vi "Motor&Controller test sequence.vi"() -> ()   [LabVIEW 2016]
uses:
  Set Save Object Dictionary.vi
  <vilib>/CANopenLib/CANOPEN.llb/CANopen SDO Create.vi
  Set mode of operation.vi
  <vilib>/CANopenLib/CANOPEN.llb/CANopen SDO Write.vi
  <vilib>/CANopenLib/CANOPEN.llb/CANopen SDO Write [STR].vi
  Get mode of operation.vi
  Set control mode.vi
  Set into drive mode.vi
  Set target speed.vi
  <vilib>/CANopenLib/CANOPEN.llb/CANopen SDO Close.vi
  <vilib>/CANopenLib/CANOPEN.llb/CANopen Interface Close.vi
panel:
  in  "OK Button":bool
  out "Mode of operation":i8(ring) items=["Induction VF – testing purposes only"=-5, "Aligning rotor position"=-4, "Current stepper – testing purposes only "=-3, "Voltage stepper – testing purposes only"=-2, "Voltage constant angle – testing purposes only"=-1, "No mode"=0, "Cyclic sync position"=8, "Cyclic sync velocity"=9, "Cyclic sync torque"=10]
  out "Error":errorcluster
  in  "Stop Button":bool
  in  "Motor Speed":i32(knob) min=0 max=1500 step=100 scale=0.0..2000.0
  in  "Motor":u8(ring) items=["Right", "Left"]
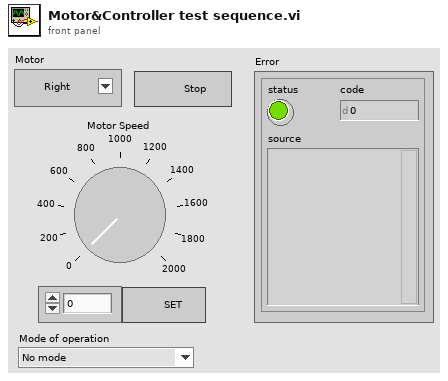
[diagram p1: front panel]
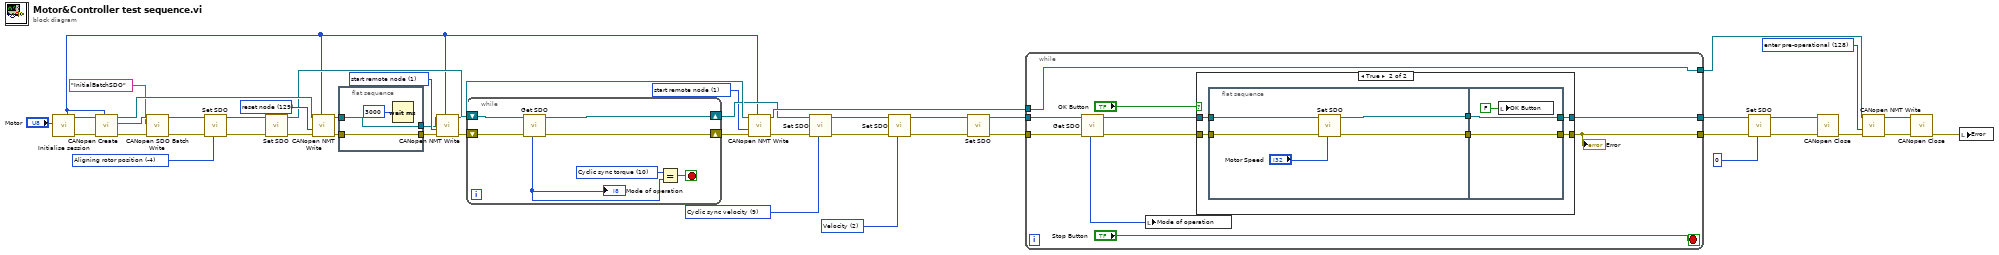
[diagram p0: block diagram]
diagram:
  w7 = u16 1 items=["start remote node"=1, "stop remote node"=2, "enter pre-operational"=128, "reset node"=129, "reset communication"=130] ("command")
  w15 = i8 9 items=["Induction VF – testing purposes only"=-5, "Aligning rotor position"=-4, "Current stepper – testing purposes only "=-3, "Voltage stepper – testing purposes only"=-2, "Voltage constant angle – testing purposes only"=-1, "No mode"=0, "Cyclic sync position"=8, "Cyclic sync velocity"=9, "Cyclic sync torque"=10] ("Mode of operation")
  w20 = u8 2 items=["Velocity"=2, "Torque"=1] ("Control Mode")
  w31 = u16 1 items=["start remote node"=1, "stop remote node"=2, "enter pre-operational"=128, "reset node"=129, "reset communication"=130] ("command")
  w32 = u16 129 items=["start remote node"=1, "stop remote node"=2, "enter pre-operational"=128, "reset node"=129, "reset communication"=130] ("command")
  w42 = u16 128 items=["start remote node"=1, "stop remote node"=2, "enter pre-operational"=128, "reset node"=129, "reset communication"=130] ("command")
  w46 = i8 -4 items=["Induction VF – testing purposes only"=-5, "Aligning rotor position"=-4, "Current stepper – testing purposes only "=-3, "Voltage stepper – testing purposes only"=-2, "Voltage constant angle – testing purposes only"=-1, "No mode"=0, "Cyclic sync position"=8, "Cyclic sync velocity"=9, "Cyclic sync torque"=10] ("Mode of operation")
  n1 = call "Initialise session.vi"("Motor"="Motor") -> ("error out"=w45:errorcluster, "interface object out"=w44:refnum<k20>, "Used Node ID"=w1:u8)  [unwired: 8 in]
  n2 = call-poly <vilib>:"CANopen Create.vi"("node-ID"=w1, "error in (no error)"=w45, "interface object in"=w44) -> ("error out"=w6:errorcluster, "SDO object out"=w3:refnum<k20>, "interface object out"=w27:refnum<k20>)  [unwired: 6 in]
  n3 = call <vilib>:"CANopen SDO Batch Write.vi"("error in (no error)"=w6, "batch SDO name"="InitialBatchSDO", "SDO object in"=w3) -> ("error out"=w5:errorcluster, "SDO object out"=w4:refnum<k20>)  [unwired: 6 in, 1 out]
  n4 = call-poly "Set SDO.vi"("Mode of operation"=w46, "error in (no error)"=w5, "SDO object in"=w4) -> ("error out"=w29:errorcluster, "SDO object out"=w30:refnum<k20>)  [unwired: 6 in, 1 out]
  n5 = call-poly "Set SDO.vi"("error in (no error)"=w29, "SDO object in"=w30) -> ("error out"=w28:errorcluster, "SDO object out"=w25:refnum<k20>)  [unwired: 7 in, 1 out]
  n6 = call <vilib>:"CANopen NMT Write.vi"("node-ID (0)"=w1, "error in (no error)"=w28, "command"=w32, "interface object in"=w27) -> ("error out"=w23:errorcluster, "interface object out"=w24:refnum<k20>)  [unwired: 6 in]
  n7 = flat-sequence {
    tunnel: w24 -> [w49]
    tunnel: w23 -> [w50]
    tunnel: [w50] -> w22
    tunnel: [w49] -> w21
    frame #0 {
      n8 = Wait (ms)(milliseconds to wait=u32 3000) -> ()  [unwired: 1 out]
    }
  }
  n9 = call <vilib>:"CANopen NMT Write.vi"("node-ID (0)"=w1, "error in (no error)"=w22, "command"=w31, "interface object in"=w21) -> ("error out"=w26:errorcluster, "interface object out"=w11:refnum<k20>)  [unwired: 6 in]
  n10 = while {
    shift-right: [w54] -> w12
    shift-left: w26 -> [w57]
    shift-right: [w55] -> w9
    shift-left: w25 -> [w56]
    stop <- w51 stop-if-true
    w53 = i8 10 items=["Induction VF – testing purposes only"=-5, "Aligning rotor position"=-4, "Current stepper – testing purposes only "=-3, "Voltage stepper – testing purposes only"=-2, "Voltage constant angle – testing purposes only"=-1, "No mode"=0, "Cyclic sync position"=8, "Cyclic sync velocity"=9, "Cyclic sync torque"=10] ("Mode of operation")
    n11 = call-poly "Get SDO.vi"("error in (no error)"=w57, "SDO object in"=w56) -> ("error out"=w54:errorcluster, "SDO object out"=w55:refnum<k20>, "Mode of operation"=w52:i8)  [unwired: 6 in, 1 out]
    "Mode of operation" <- w52
    n12 = Equal?(x=w53, y=w52) -> (x = y?=w51:bool)
  }
  n13 = call <vilib>:"CANopen NMT Write.vi"("node-ID (0)"=w1, "error in (no error)"=w12, "command"=w7, "interface object in"=w11) -> ("error out"=w8:errorcluster, "interface object out"=w10:refnum<k20>)  [unwired: 6 in]
  n14 = call-poly "Set SDO.vi"("Mode of operation"=w15, "error in (no error)"=w8, "SDO object in"=w9) -> ("error out"=w18:errorcluster, "SDO object out"=w19:refnum<k20>)  [unwired: 6 in, 1 out]
  n15 = call-poly "Set SDO.vi"("Control Mode"=w20, "error in (no error)"=w18, "SDO object in"=w19) -> ("error out"=w16:errorcluster, "SDO object out"=w17:refnum<k20>)  [unwired: 6 in, 1 out]
  n16 = call-poly "Set SDO.vi"("error in (no error)"=w16, "SDO object in"=w17) -> ("error out"=w13:errorcluster, "SDO object out"=w14:refnum<k20>)  [unwired: 8 in]
  n17 = while {
    tunnel: [w66] -> w41
    tunnel: [w64] -> w40
    tunnel: w10 -> [w65]
    tunnel: [w65] -> w39
    tunnel: w14 -> [w59]
    tunnel: w13 -> [w58]
    stop <- "Stop Button" stop-if-true
    n18 = call-poly "Get SDO.vi"("error in (no error)"=w58, "SDO object in"=w59) -> ("error out"=w60:errorcluster, "SDO object out"=w61:refnum<k20>, "Mode of operation"=w62:i8)  [unwired: 6 in, 1 out]
    n19 = local write "Mode of operation"(w62) -> ()
    n20 = case shown="True" "OK Button" {
      tunnel: [w69 w75] -> w66
      tunnel: [w68 w74] -> w64
      tunnel: w61 -> [w69 w71]
      tunnel: w60 -> [w68 w70]
      frame False {
      }
      frame True {
        n21 = flat-sequence {
          tunnel: [w80] -> w73
          tunnel: [w79] -> w72
          tunnel: w71 -> [w77]
          tunnel: w70 -> [w76]
          tunnel: [w82] -> w74
          tunnel: [w83] -> w75
          tunnel: w73 -> [w83]
          tunnel: w72 -> [w82]
          frame #0 {
            n22 = call-poly "Set SDO.vi"("Speed"="Motor Speed", "error in (no error)"=w76, "SDO object in"=w77) -> ("error out"=w79:errorcluster, "SDO object out"=w80:refnum<k20>)  [unwired: 6 in, 1 out]
          }
          frame #1 {
            n23 = local write "OK Button"(FALSE ("OK Button")) -> ()
          }
        }
      }
    }
    "Error" <- w64
  }
  n24 = call-poly "Set SDO.vi"("Speed"=0, "error in (no error)"=w40, "SDO object in"=w41) -> ("error out"=w38:errorcluster, "SDO object out"=w37:refnum<k20>)  [unwired: 6 in, 1 out]
  n25 = call-poly <vilib>:"CANopen Close.vi"("error in (no error)"=w38, "SDO object in"=w37) -> ("error out"=w36:errorcluster)  [unwired: 9 in]
  n26 = call <vilib>:"CANopen NMT Write.vi"("error in (no error)"=w36, "command"=w42, "interface object in"=w39) -> ("error out"=w34:errorcluster, "interface object out"=w35:refnum<k20>)  [unwired: 7 in]
  n27 = call-poly <vilib>:"CANopen Close.vi"("error in (no error)"=w34, "interface object in"=w35) -> ("error out"=w33:errorcluster)  [unwired: 9 in]
  n28 = local write "Error"(w33) -> ()
